vi "Comm Parms.vi"() -> (1 "Com Parms Out":T1={"Port"="COM3", "Baud Rate"=38400, "Data Bits"=8, "Parity"=0, "Stop Bits"=10, "Flow Control"=0} {"Flow Control" items=["None"=0, "XON/XOFF"=1, "RTS/CTS"=2, "DTR/DSR"=4]; "Stop Bits" items=["1.0"=10, "1.5"=15, "2.0"=20]; "Parity" items=["None", "Odd", "Even", "Mark", "Space"]; "Data Bits" min=5 max=8 step=1})   [LabVIEW 2012]
uses:
  Type Defs/Comm Settings.ctl
panel:
  in  "Return":bool
  in  "Com Parms":T1={"Port"="COM3", "Baud Rate"=38400, "Data Bits"=8, "Parity"=0, "Stop Bits"=10, "Flow Control"=0} {"Flow Control" items=["None"=0, "XON/XOFF"=1, "RTS/CTS"=2, "DTR/DSR"=4]; "Stop Bits" items=["1.0"=10, "1.5"=15, "2.0"=20]; "Parity" items=["None", "Odd", "Even", "Mark", "Space"]; "Data Bits" min=5 max=8 step=1}
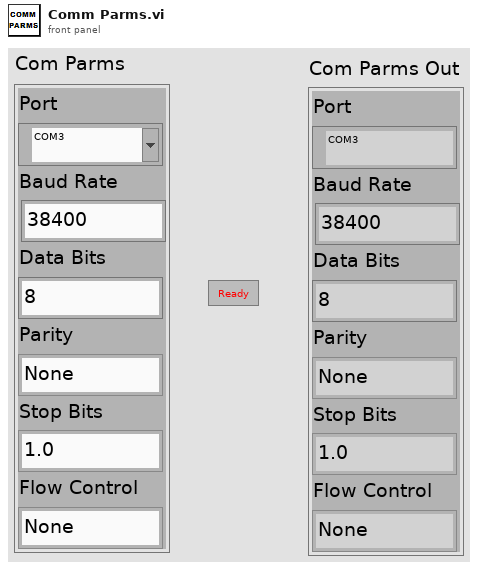
[diagram p1: front panel]
types:
  T1 = typedef "Comm Settings.ctl" = cluster{"Port":refnum<visa-resource-name>, "Baud Rate":u32, "Data Bits":u16, "Parity":u16, "Stop Bits":u16, "Flow Control":u16}
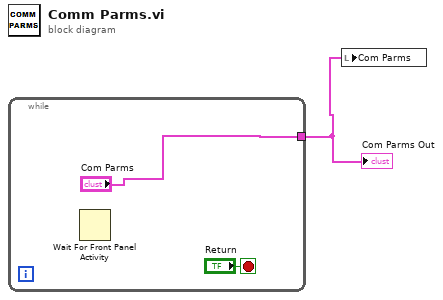
[diagram p0: block diagram]
diagram:
  n1 = while {
    tunnel: ["Com Parms"] -> w1
    stop <- "Return" stop-if-true
    n2 = Wait For Front Panel Activity() -> ()  [unwired: 3 in, 1 out]
  }
  "Com Parms Out" <- w1
  n3 = local write "Com Parms"(w1) -> ()
